vi "receive header message.vi"(8 "error in (no error)":errorcluster, 11 "Channel in":refnum<class "SPARC4_Channel.lvclass">) -> (0 "error out":errorcluster, 3 "Channel out":refnum<class "SPARC4_Channel.lvclass">)   [LabVIEW 2018, in "SPARC4_Channel.lvclass"]
uses:
  SPARC4_Channel.lvclass
  SPARC4_Channel.lvclass/SPARC4_Channel.ctl
  Server/Server.lvclass
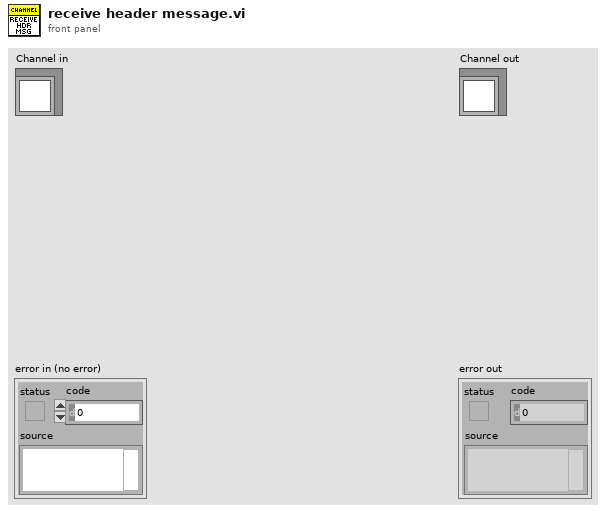
[diagram p1: front panel]
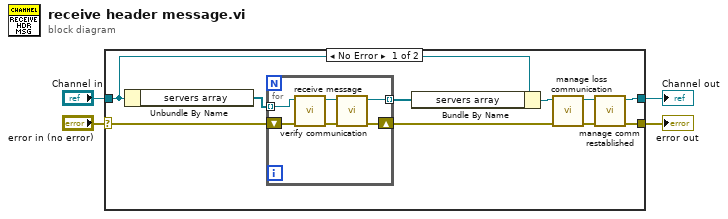
[diagram p0: block diagram]
diagram:
  n1 = case shown="No Error" "error in (no error)" {
    selector: "error in (no error)" -> [w5 w22]
    tunnel: [w10 w22] -> w3
    tunnel: [w11 w21] -> w1
    tunnel: "Channel in" -> [w14 w21]
    frame No Error {
      n2 = Unbundle By Name(w14) -> ("servers array"=w8:refnum<class "Server.lvclass">[])
      n3 = for {
        shift-right: [w16] -> w6
        shift-left: w5 -> [w19]
        tunnel: [w15] -> w7 mode=indexing
        tunnel: w8 -> [w20] mode=indexing
        n4 = call "receive message.vi"("error in (no error)"=w19, "Server in"=w20) -> ("error out"=w17:errorcluster, "Server out"=w18:refnum<class "Server.lvclass">)  [unwired: 8 in]
        n5 = call "verify communication.vi"("error in (no error)"=w17, "Server in"=w18) -> ("error out"=w16:errorcluster, "Server out"=w15:refnum<class "Server.lvclass">)  [unwired: 8 in]
      }
      n6 = Bundle By Name(cluster=w14, "servers array"=w7) -> (w13:refnum<class "SPARC4_Channel.lvclass">)
      n7 = call "manage loss communication.vi"("error in (no error)"=w6, "Channel in"=w13) -> ("error out"=w9:errorcluster, "Channel out"=w12:refnum<class "SPARC4_Channel.lvclass">)  [unwired: 8 in]
      n8 = call "manage comm restablished.vi"("error in (no error)"=w9, "Channel in"=w12) -> ("error out"=w10:errorcluster, "Channel out"=w11:refnum<class "SPARC4_Channel.lvclass">)  [unwired: 8 in]
    }
    frame Error {
    }
  }
  "error out" <- w3
  "Channel out" <- w1
